vi "Unflatten to PDU.vi"(8 "error in":errorcluster, 10 "ELAN data unit data":u8[](array[numeric])) -> (0 "error out":errorcluster, 3 "ELAN data unit out":refnum<class "ELAN PDU.lvclass">)   [LabVIEW 2021, in "ELAN PDU.lvclass"]
uses:
  ELAN PDU.lvclass
  ELAN PDU.lvclass/ELAN PDU.ctl
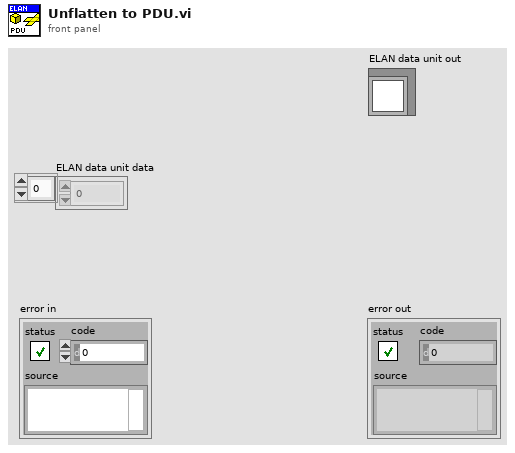
[diagram p1: front panel]
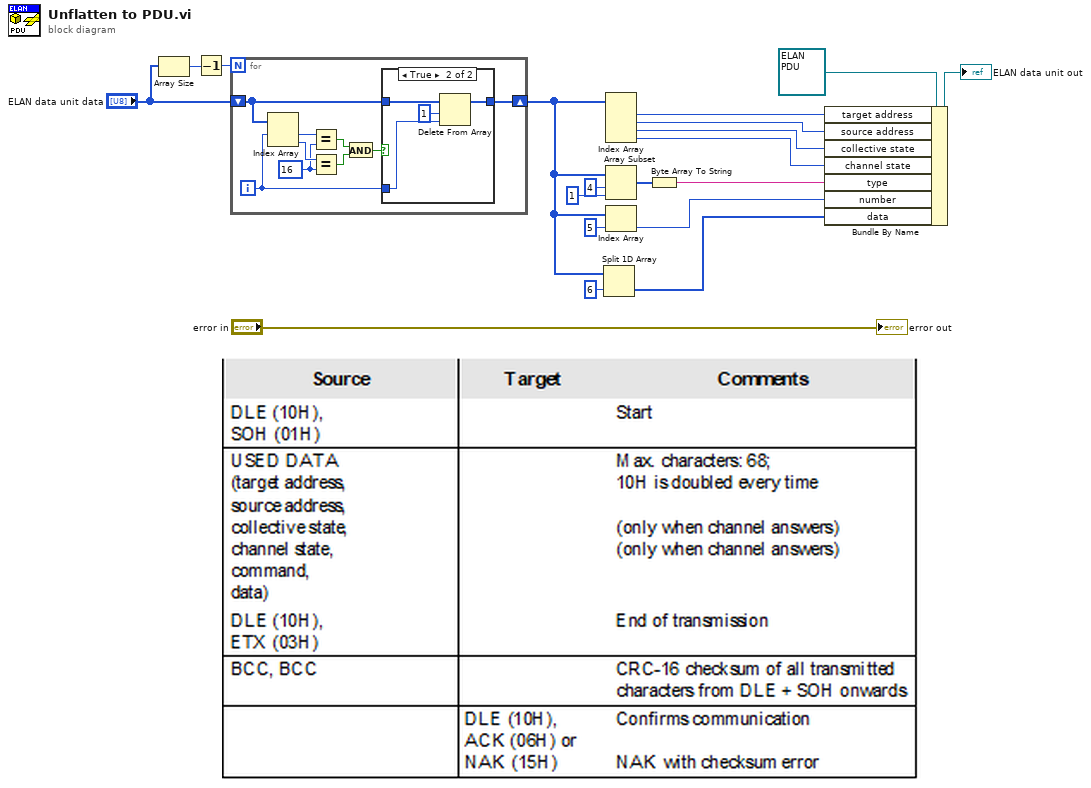
[diagram p0: block diagram]
diagram:
  n1 = Array Size(array="ELAN data unit data") -> (size(s)=w5:i32)
  n2 = Decrement(x=w5) -> (x-1=w6:i32)
  n3 = for {
    N: w6 -> [_]
    shift-right: [w26] -> w3
    shift-left: "ELAN data unit data" -> [w20]
    i -> [w27]
    w23 = u8 16 ("y")
    n4 = Index Array(array=w20, index #1=w27) -> (element #1=w28:u8, element #2=w24:u8)  [unwired: 1 in]
    n5 = Equal?(x=w28, y=w23) -> (x = y?=w25:bool)
    n6 = Equal?(x=w24, y=w23) -> (x = y?=w21:bool)
    n7 = And(x=w25, y=w21) -> (x .and. y?=w22:bool)
    n8 = case shown="True" w22 {
      tunnel: w20 -> [w29 w33]
      tunnel: w27 -> [_ w31]
      tunnel: [w29 w32] -> w26
      frame False {
      }
      frame True {
        n9 = Delete From Array(array=w33, length=1, index=w31) -> (array with subset deleted=w32:u8[])  [unwired: 1 out]
      }
    }
  }
  n10 = Split 1D Array(array=w3, index=6) -> (second subarray=w2:u8[])  [unwired: 1 out]
  n11 = Index Array(array=w3) -> (element #1=w17:u8, element #2=w16:u8, element #3=w8:u8, element #4=w7:u8)  [unwired: 4 in]
  n12 = Array Subset(array=w3, index=4, length=1) -> (w13:u8[])
  n13 = Index Array(array=w3, index=5) -> (element=w10:u8)
  n14 = Byte Array To String(unsigned byte array=w13) -> (string=w11:string)
  n15 = Bundle By Name(cluster=refnum<class "ELAN PDU.lvclass"> refnum ("ELAN data unit"), "target address"=w17, "source address"=w16, "collective state"=w8, "channel state"=w7, "type"=w11, "number"=w10, "data"=w2) -> (→"ELAN data unit out":refnum<class "ELAN PDU.lvclass">)
  "error out" <- "error in"
